vi "Action to String.vi"(8 "error in (no error)":errorcluster, 9 "Action Data":string[][](array[string]), 10 "String Format":string, 11 "Action Name":string) -> (0 "error out":errorcluster, 3 "String":string)   [LabVIEW 2016, in "Hardware.lvlib" / "Motions.lvlib" / "Motions.lvclass"]
uses:
  <userlib>/Common Components/Hardware/Abstract System/Motions/Motions/Motions.lvclass
panel:
  # "path"
  # "data"
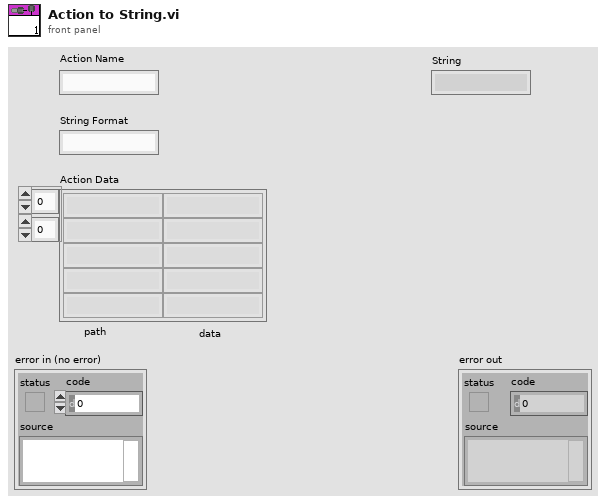
[diagram p1: front panel]
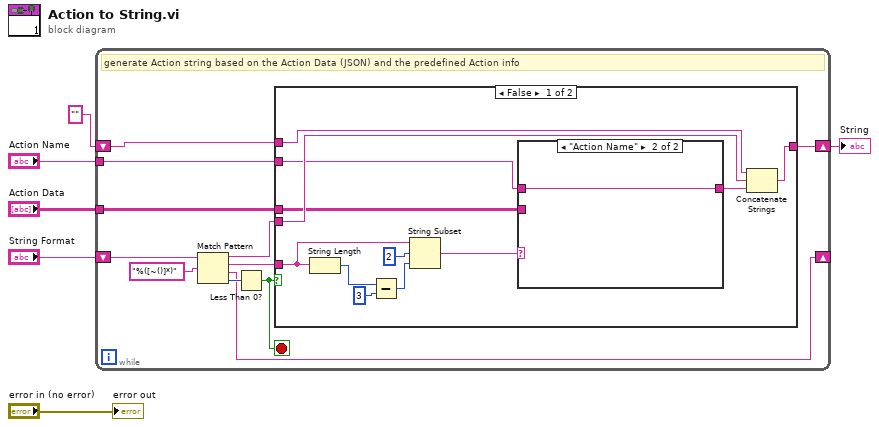
[diagram p0: block diagram]
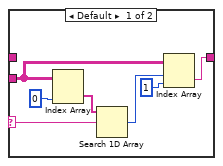
[diagram p2: hidden frame]
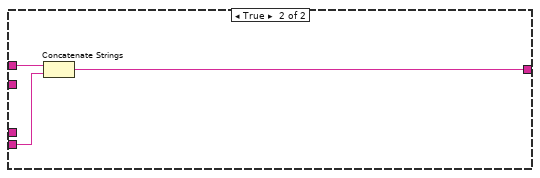
[diagram p3: hidden frame]
diagram:
  n1 = while {
    shift-right: [w12] -> w1
    shift-left: "" -> [w14]
    tunnel: "Action Name" -> [w10]
    shift-right: [w9] -> _
    shift-left: "String Format" -> [w17]
    tunnel: "Action Data" -> [w7]
    stop <- w8 stop-if-true
    # "generate Action string based on the Action Data (JSON) and the predefined Action info"
    n2 = Match Pattern(string=w17, regular expression="%([~()]*)") -> (before substring=w13:string, match substring=w11:string, after substring=w9:string, offset past match=w15:i32)  [unwired: 1 in]
    n3 = Less Than 0?(x=w15) -> (x < 0?=w8:bool)
    n4 = case shown="False" w8 {
      tunnel: w14 -> [w29 w40]
      tunnel: w13 -> [w28 w39]
      tunnel: [w27 w38] -> w12
      tunnel: w11 -> [w25 _]
      tunnel: w10 -> [w20 _]
      tunnel: w7 -> [w18 _]
      frame False {
        n5 = String Length(string=w25) -> (length=w24:i32)
        n6 = Subtract(x=w24, y=3) -> (x-y=w22:i32)
        n7 = String Subset(string=w25, offset (0)=2, length (rest)=w22) -> (substring=w21:string)
        n8 = case shown="\"Action Name\"" w21 {
          selector: w21 -> [w34 _]
          tunnel: w20 -> [_ w37]
          tunnel: [w30 w37] -> w19
          tunnel: w18 -> [w33 _]
          frame Default {
            n9 = Index Array(array=w33, index (col)=0 ("disabled index (col)")) -> (element=w35:string[])  [unwired: 1 in]
            n10 = Search 1D Array(1D array=w35, element=w34) -> (index of element=w32:i32)  [unwired: 1 in]
            n11 = Index Array(array=w33, index (row)=w32, index (col)=1 ("disabled index (col)")) -> (element=w30:string)
          }
          frame "Action Name" {
          }
        }
        n12 = Concatenate Strings(w29, w28, w19) -> (w27:string)
      }
      frame True {
        n13 = Concatenate Strings(w40, w39) -> (w38:string)
      }
    }
  }
  "String" <- w1
  "error out" <- "error in (no error)"
